vi "writeToClient.vi"(8 "error in (no error)":errorcluster, 10 "packetConnID":T1, 11 "tcpServer in":refnum<class "TcpServer.lvclass">) -> (0 "error out":errorcluster, 3 "tcpServer out":refnum<class "TcpServer.lvclass">)   [LabVIEW 2018, in "TcpServer.lvclass"]
doc: "Write packet to the TCP Client."
uses:
  TcpServer.lvclass
  typedef/packetConnIDTypeDef.ctl
  TcpServer.lvclass/TcpServer.ctl
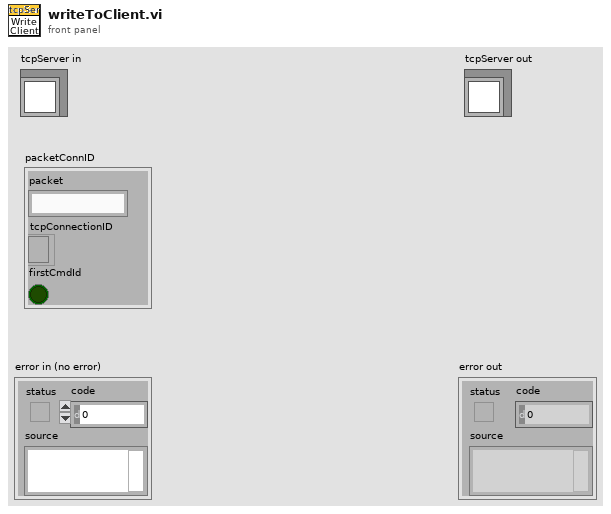
[diagram p1: front panel]
types:
  T1 = typedef "TcpServer.lvclass/packetConnIDTypeDef.ctl" = cluster{"packet":string, "tcpConnectionID":refnum<k5>, "firstCmdId":bool}
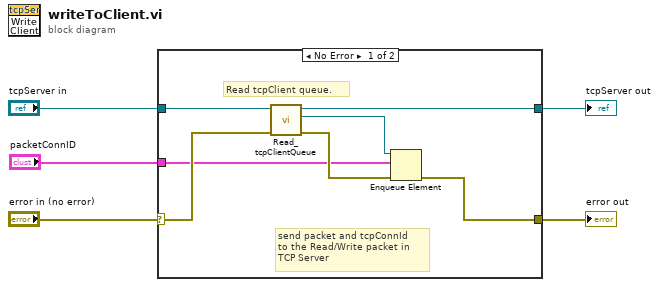
[diagram p0: block diagram]
diagram:
  n1 = case shown="No Error" "error in (no error)" {
    selector: "error in (no error)" -> [w8 w14]
    tunnel: [w7 w14] -> w4
    tunnel: [w9 w13] -> w2
    tunnel: "tcpServer in" -> [w10 w13]
    tunnel: "packetConnID" -> [w6 _]
    frame No Error {
      # "send packet and tcpConnId\nto the Read/Write packet in \nTCP Server"
      # "Read tcpClient queue."
      n2 = call "Read_tcpClientQueue.vi"("error in (no error)"=w8, "tcpServer in"=w10) -> ("error out"=w11:errorcluster, "tcpClientQueue"=w12:refnum<queue>, "tcpServer out"=w9:refnum<class "TcpServer.lvclass">)  [unwired: 7 in]
      n3 = Enqueue Element(queue=w12, element=w6, error in (no error)=w11) -> (error out=w7:errorcluster)  [unwired: 1 in, 2 out]
    }
    frame Error {
    }
  }
  "error out" <- w4
  "tcpServer out" <- w2
